vi "MesaurementProcedure.vi"(8 "error in (no error)":errorcluster) -> (0 "error out":errorcluster)   [LabVIEW 2013]
uses:
  Utilities/controls/ctlSeqFNs_PI_SysNr.ctl
  Camera/lib/atmcd32d.llb/Error Code Enum typedef.ctl
  <vilib>/DAQmx/write.llb/DAQmx Write (Analog DBL 1Chan 1Samp).vi
  <vilib>/DAQmx/read.llb/DAQmx Read (Analog DBL 1Chan 1Samp).vi
  Variables/GlobalSetGetPixelOfRoi.vi
  Variables/GlobalSetConfigurationPhysikalInstruments.vi
  Variables/ccdChipPixels.vi
  Variables/GlobalSetGetConfigureCamera.vi
  Variables/SavPath.vi
  Variables/GlobalDevice.vi
  Variables/MesaurementModus.vi
  Variables/ScanrangeY.vi
  Variables/ScanrangeX.vi
  <vilib>/DAQmx/create/channels.llb/DAQmx Create Channel (CO-Pulse Generation-Frequency).vi
  <vilib>/DAQmx/configure/trigger.llb/DAQmx Start Trigger (Digital Edge).vi
  <vilib>/DAQmx/configure/timing.llb/DAQmx Timing (Implicit).vi
  <vilib>/DAQmx/create/channels.llb/DAQmx Create Channel (AI-Voltage-Basic).vi
  <vilib>/DAQmx/create/channels.llb/DAQmx Create Channel (AO-Voltage-Basic).vi
  <vilib>/DAQmx/miscellaneous.llb/DAQmx Fill In Error Info.vi
  Variables/GlobalMesaurementOut.vi
  <resource>/objmgr/daqmx.rc
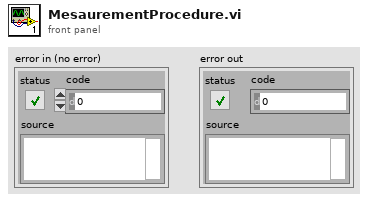
[diagram p1: front panel]
types:
  T1 = typedef "ctlSeqFNs_PI_SysNr.ctl" = enum16{"Zero", "E517", "E710"}
  T2 = typedef "Error Code Enum typedef.ctl" = enum32{"N/A (0)", "DRV_ERROR_CODES", "DRV_SUCCESS", "DRV_VXDNOTINSTALLED", "DRV_ERROR_SCAN", "DRV_ERROR_CHECK_SUM", "DRV_ERROR_FILELOAD", "DRV_UNKNOWN_FUNC", "DRV_ERROR_VXD_INIT", "DRV_ERROR_ADDRESS", "DRV_ERROR_PAGELOCK", "DRV_ERROR_PAGEUNLOCK", "DRV_ERROR_BOARDTEST", "DRV_ERROR_ACK", "DRV_ERROR_UP_FIFO", "DRV_ERROR_PATTERN", "N/A (16)", "DRV_ACQUISITION_ERRORS", "DRV_ACQ_BUFFER", "DRV_ACQ_DOWNFIFO_FULL", "DRV_PROC_UNKONWN_INSTRUCTION", "DRV_ILLEGAL_OP_CODE", "DRV_KINETIC_TIME_NOT_MET", "DRV_ACCUM_TIME_NOT_MET", "DRV_NO_NEW_DATA", "N/A (25)", "DRV_SPOOLERROR", "N/A (27)", "N/A (28)", "N/A (29)", "N/A (30)", "N/A (31)", "N/A (32)", "DRV_TEMPERATURE_CODES", "DRV_TEMPERATURE_OFF", "DRV_TEMPERATURE_NOT_STABILIZED", "DRV_TEMPERATURE_STABILIZED", "DRV_TEMPERATURE_NOT_REACHED", "DRV_TEMPERATURE_OUT_RANGE", "DRV_TEMPERATURE_NOT_SUPPORTED", "DRV_TEMPERATURE_DRIFT", "N/A (41)", "N/A (42)", "N/A (43)", "N/A (44)", "N/A (45)", "N/A (46)", "N/A (47)", "N/A (48)", "DRV_GENERAL_ERRORS", "DRV_INVALID_AUX", "DRV_COF_NOTLOADED", "DRV_FPGAPROG", "DRV_FLEXERROR", "DRV_GPIBERROR", "N/A (55)", "N/A (56)", "N/A (57)", "N/A (58)", "N/A (59)", "N/A (60)", "N/A (61)", "N/A (62)", "N/A (63)", "DRV_DATATYPE", "DRV_DRIVER_ERRORS", "DRV_P1INVALID", "DRV_P2INVALID", "DRV_P3INVALID", "DRV_P4INVALID", "DRV_INIERROR", "DRV_COFERROR", "DRV_ACQUIRING", "DRV_IDLE", "DRV_TEMPCYCLE", "DRV_NOT_INITIALIZED", "DRV_P5INVALID", "DRV_P6INVALID", "DRV_INVALID_MODE", "DRV_INVALID_FILTER", "DRV_I2CERRORS", "DRV_I2CDEVNOTFOUND", "DRV_I2CTIMEOUT", "DRV_P7INVALID", "N/A (84)", "N/A (85)", "N/A (86)", "N/A (87)", "N/A (88)", "N/A (89)", "DRV_IOCERROR", "DRV_VRMVERSIONERROR"}
  T3 = cluster{"Conn. Axes scanner[0]":string, "Conn. Axes scanner[1]":string, "Conn. Axes scanner[2]":string}
  T4 = enum16{"open", "replace", "create", "open or create", "replace or create", "replace or create with confirmation"}
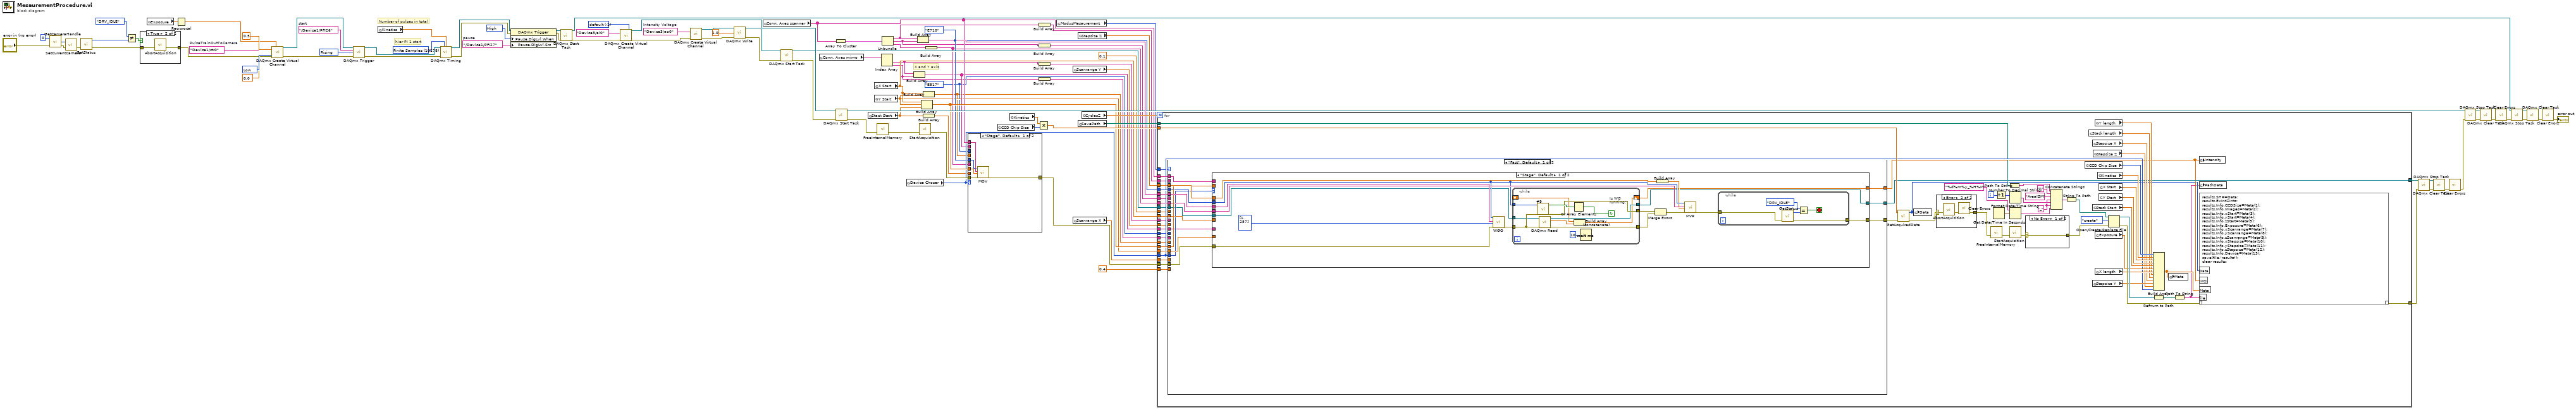
[diagram p0: block diagram]
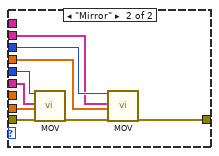
[diagram p2: hidden frame]
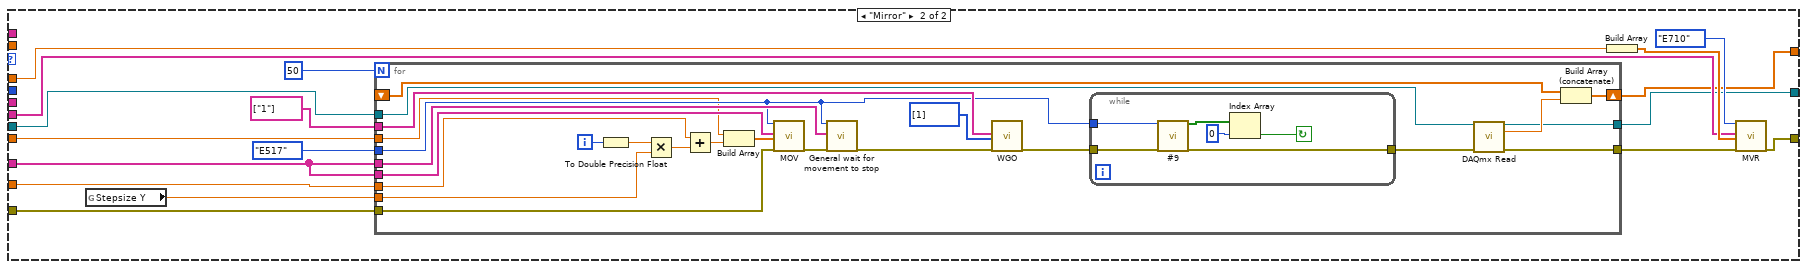
[diagram p3: hidden frame]
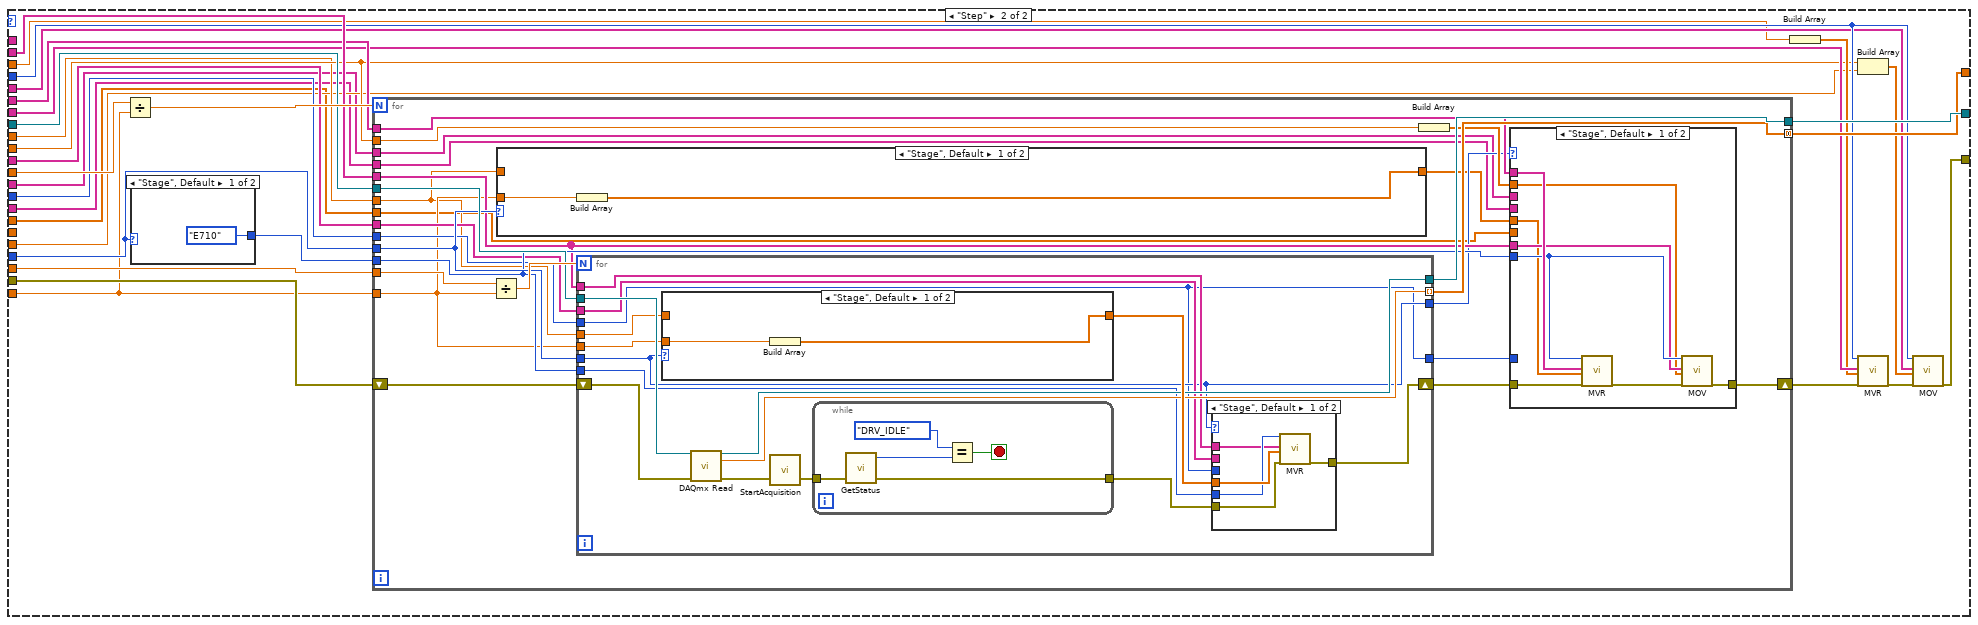
[diagram p4: hidden frame]
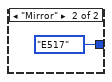
[diagram p5: hidden frame]
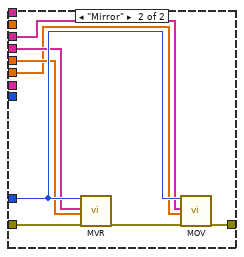
[diagram p6: hidden frame]
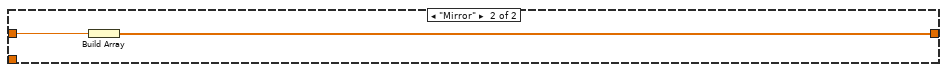
[diagram p7: hidden frame]
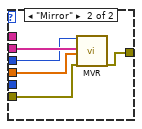
[diagram p8: hidden frame]
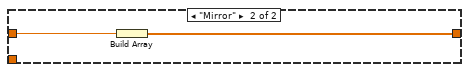
[diagram p9: hidden frame]
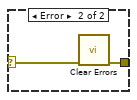
[diagram p11: hidden frame]
diagram:
  w10 = tag "/Device1/PFI26"  # start
  w11 = tag "/Device1/PFI27"  # pause
  w16 = 10192 items=["High"=10192, "Low"=10214] ("Pause.DigLvl.When")
  w21 = 10280 items=["Rising"=10280, "Falling"=10171] ("Trigger Edge")
  w17 = tag "Device1/ctr0"  # PulseTrainOutToCamera
  w27 = 10214 items=["High"=10192, "Low"=10214] ("Idle State")
  w28 = 10178 items=["Finite Samples"=10178, "Continuous Samples"=10123] ("sample mode")
  w36 = ctlSeqFNs_PI_SysNr."E517" ("DeviceNr.")
  w76 = tag "Device3/ao0"  # Intensity Voltage
  w78 = -1 items=["default"=-1, "RSE"=10083, "NRSE"=10078, "Differential"=10106, "Pseudodifferential"=12529] ("input terminal configuration")
  w51 = ctlSeqFNs_PI_SysNr."E710" ("DeviceNr.")
  # "Number of pulses in total"
  # "hier PI 1 start"
  # "X and Y axis"
  n1 = call "GetCameraHandle.vi"("error in (no error)"="error in (no error)", "cameraIndex"=0) -> ("error out"=w86:errorcluster, "cameraHandle"=w85:i32)  [unwired: 1 in, 1 out]
  n2 = call "SetCurrentCamera.vi"("error in (no error)"=w86, "cameraHandle"=w85) -> ("error out"=w87:errorcluster)  [unwired: 1 out]
  n3 = call "GetStatus.vi"("error in (no error)"=w87) -> ("error out"=w92:errorcluster, "status"=w89:T2)  [unwired: 2 in, 1 out]
  n4 = Not Equal?(x=Error_Code_Enum_typedef."DRV_IDLE" ("status"), y=w89) -> (x != y?=w91:bool)
  n5 = case shown="True" w91 {
    tunnel: w92 -> [w99 w101]
    tunnel: [w99 w100] -> w19
    frame False {
    }
    frame True {
      n6 = call "AbortAcquisition.vi"("error in (no error)"=w101) -> ("error out"=w100:errorcluster)  [unwired: 1 in, 1 out]
    }
  }
  n7 = global read "GlobalSetGetConfigureCamera.vi" "Exposure"() -> (w2:sgl)
  n8 = Reciprocal(x=w2) -> (1/x=w3:sgl)
  n9 = call-poly <vilib>:"DAQmx Create Virtual Channel.vi"("frequency"=w3, "duty cycle"=0.5 ("Duty Cycle"), "counter"=w17, "error in"=w19, "idle state"=w27, "initial delay"=0.0) -> ("task out"=w24:refnum<k21>, "error out"=w22:errorcluster)  [unwired: 8 in]
  n10 = call-poly <vilib>:"DAQmx Trigger.vi"("task/channels in"=w24, "source"=w10, "edge"=w21, "error in"=w22) -> ("task out"=w20:refnum<k21>, "error out"=w23:errorcluster)  [unwired: 10 in]
  n11 = global read "GlobalSetGetConfigureCamera.vi" "Kinetics"() -> (w1:sgl)
  n12 = call-poly <vilib>:"DAQmx Timing.vi"("task/channels in"=w20, "sample mode"=w28, "samples per channel"=w1, "error in"=w23) -> ("task out"=w13:refnum<k21>, "error out"=w15:errorcluster)  [unwired: 10 in]
  n13 = property class="DAQmx Trigger"(reference=w13, error in=w15, "Pause.DigLvl.When"=w16, "Pause.DigLvl.Src"=w11) -> (reference out=w12:refnum<k21>, error out=w14:errorcluster)
  n14 = call <vilib>:"DAQmx Start Task.vi"("task/channels in"=w12, "error in"=w14) -> ("task out"=w4:refnum<k21>, "error out"=w18:errorcluster)  [unwired: 12 in]
  n15 = call-poly <vilib>:"DAQmx Create Virtual Channel.vi"("input terminal configuration"=w78, "physical channels"=tag "Device3/ai0", "error in"=w18) -> ("task out"=w67:refnum<k21>, "error out"=w68:errorcluster)  [unwired: 11 in]
  n16 = call-poly <vilib>:"DAQmx Create Virtual Channel.vi"("physical channels"=w76, "error in"=w68) -> ("task out"=w75:refnum<k21>, "error out"=w77:errorcluster)  [unwired: 12 in]
  n17 = call-poly <vilib>:"DAQmx Write.vi"("task/channels in"=w75, "data"=1.0, "error in"=w77) -> ("task out"=w71:refnum<k21>, "error out"=w73:errorcluster)  [unwired: 10 in, 1 out]
  n18 = global read "GlobalSetConfigurationPhysikalInstruments.vi" "Conn. Axes scanner"() -> (w52:string[])
  n19 = call <vilib>:"DAQmx Start Task.vi"("task/channels in"=w67, "error in"=w73) -> ("task out"=w66:refnum<k21>, "error out"=w72:errorcluster)  [unwired: 12 in]
  n20 = global read "GlobalSetConfigurationPhysikalInstruments.vi" "Conn. Axes mirrro"() -> (w50:string[])
  n21 = Array To Cluster(array=w52) -> (cluster=w84:T3)
  n22 = call <vilib>:"DAQmx Start Task.vi"("task/channels in"=w71, "error in"=w72) -> ("task out"=w61:refnum<k21>, "error out"=w70:errorcluster)  [unwired: 12 in]
  n23 = global read "GlobalSetGetPixelOfRoi.vi" "Stack Start"() -> (w44:dbl)
  n24 = global read "GlobalSetGetPixelOfRoi.vi" "X Start"() -> (w40:dbl)
  n25 = global read "GlobalSetGetPixelOfRoi.vi" "Y Start"() -> (w39:dbl)
  n26 = call "FreeInternalMemory.vi"("error in (no error)"=w70) -> ("error out"=w93:errorcluster)  [unwired: 1 in, 1 out]
  n27 = Index Array(array=w50) -> (element #1=w38:string, element #2=w34:string)  [unwired: 2 in]
  n28 = Unbundle(w84) -> ("Conn. Axes scanner[0]"=w49:string, "Conn. Axes scanner[1]"=w47:string, "Conn. Axes scanner[2]"=w83:string)
  n29 = global read "GlobalDevice.vi" "Device Choser"() -> (w45:enum32{"Stage", "Mirror"})
  n30 = Build Array(w38, w34) -> (w41:string[])
  n31 = Build Array(w49, w47) -> (w82:string[])
  n32 = call "StartAcquisition.vi"("error in (no error)"=w93) -> ("error out"=w54:errorcluster)  [unwired: 1 in, 1 out]
  n33 = Build Array(w40, w39, w44) -> (w53:dbl[])
  n34 = Build Array(w40, w39) -> (w32:dbl[])
  n35 = Build Array(w44) -> (w43:dbl[])
  n36 = Build Array(w83) -> (w42:string[])
  n37 = case shown="\"Stage\", Default" w45 {
    tunnel: [w106 w115] -> w55
    tunnel: w54 -> [w105 w113]
    tunnel: w53 -> [w104 _]
    tunnel: w52 -> [w103 _]
    tunnel: w51 -> [w102 w110]
    tunnel: w43 -> [_ w112]
    tunnel: w42 -> [_ w111]
    tunnel: w36 -> [_ w109]
    tunnel: w41 -> [_ w108]
    tunnel: w32 -> [_ w107]
    frame "Stage", Default {
      n38 = call "MOV.vi"("System no."=w102, "Axes to move"=w103, "Position values"=w104, "error in"=w105) -> ("error out"=w106:errorcluster)  [unwired: 1 in, 14 out]
    }
    frame "Mirror" {
      n39 = call "MOV.vi"("System no."=w110, "Axes to move"=w111, "Position values"=w112, "error in"=w113) -> ("error out"=w114:errorcluster)  [unwired: 1 in, 14 out]
      n40 = call "MOV.vi"("System no."=w109, "Axes to move"=w108, "Position values"=w107, "error in"=w114) -> ("error out"=w115:errorcluster)  [unwired: 1 in, 14 out]
    }
  }
  n41 = global read "ccdChipPixels.vi" "CCD Chip Size"() -> (w96:i32)
  n42 = global read "GlobalSetGetConfigureCamera.vi" "Kinetics"() -> (w97:sgl)
  n43 = Multiply(x=w97, y=w96) -> (x*y=w94:sgl)
  n44 = Build Array(w49) -> (w48:string[])
  n45 = Build Array(w47) -> (w46:string[])
  n46 = Build Array(w38) -> (w37:string[])
  n47 = Build Array(w34) -> (w33:string[])
  n48 = global read "MesaurementModus.vi" "ModusMesaurement"() -> (w30:enum32{"Fast", "Step"})
  n49 = global read "ScanrangeY.vi" "Scanrange Y"() -> (w56:dbl)
  n50 = global read "ScanrangeX.vi" "Scanrange X"() -> (w57:dbl)
  n51 = global read "GlobalSetGetPixelOfRoi.vi" "Stepsize Z"() -> (w31:dbl)
  n52 = global read "SavPath.vi" "SavePath"() -> (w95:path)
  n53 = global read "GlobalSetGetPixelOfRoi.vi" "CyclesZ"() -> (w98:dbl)
  n54 = for {
    N: w98 -> [_]
    tunnel: w52 -> [w180]
    tunnel: w31 -> [w179]
    tunnel: w82 -> [w178]
    tunnel: w53 -> [w177]
    tunnel: w42 -> [w176]
    tunnel: w51 -> [w175]
    tunnel: w94 -> [w174]
    tunnel: w95 -> [w120]
    tunnel: [w173] -> w63
    tunnel: w55 -> [w172]
    tunnel: w39 -> [w139]
    tunnel: w40 -> [w138]
    tunnel: w45 -> [w136]
    tunnel: w66 -> [w134]
    tunnel: [w133] -> w65
    tunnel: w30 -> [w132]
    tunnel: w57 -> [w130]
    tunnel: w56 -> [w131]
    tunnel: w41 -> [w129]
    tunnel: w48 -> [w128]
    tunnel: w46 -> [w127]
    tunnel: w37 -> [w126]
    tunnel: w36 -> [w125]
    tunnel: 0.1 -> [w124]
    tunnel: 0.4 -> [w123]
    tunnel: w33 -> [w122]
    tunnel: w32 -> [w121]
    i -> [w137]
    w155 = "_" ("string")
    n55 = case shown="\"Fast\", Default" w132 {
      tunnel: w180 -> [w195 _]
      tunnel: w179 -> [w194 w276]
      tunnel: w178 -> [w193 w287]
      tunnel: w177 -> [w192 _]
      tunnel: w176 -> [w191 w292]
      tunnel: w175 -> [w190 w288]
      tunnel: w172 -> [w189 w301]
      tunnel: [w188 w289] -> w171
      tunnel: w139 -> [w187 w280]
      tunnel: w138 -> [w186 w285]
      tunnel: w136 -> [w185 w295]
      tunnel: w134 -> [w184 w299]
      tunnel: [w183 w298] -> w133
      tunnel: [w182 w297] -> w119
      tunnel: w131 -> [_ w300]
      tunnel: w130 -> [_ w303]
      tunnel: w129 -> [w181 w278]
      tunnel: w128 -> [_ w294]
      tunnel: w127 -> [_ w293]
      tunnel: w126 -> [_ w284]
      tunnel: w125 -> [_ w283]
      tunnel: w124 -> [_ w282]
      tunnel: w123 -> [_ w281]
      tunnel: w122 -> [_ w279]
      tunnel: w121 -> [_ w277]
      frame "Fast", Default {
        n56 = case shown="\"Stage\", Default" w185 {
          tunnel: w195 -> [_ _]
          tunnel: w194 -> [w211 w236]
          tunnel: w193 -> [w210 _]
          tunnel: w192 -> [_ _]
          tunnel: w191 -> [w209 w234]
          tunnel: w190 -> [w208 _]
          tunnel: w189 -> [w196 w239]
          tunnel: [w203 w238] -> w188
          tunnel: w187 -> [_ w241]
          tunnel: w186 -> [_ w240]
          tunnel: [w199 w232] -> w182
          tunnel: w184 -> [w198 w231]
          tunnel: [w197 w230] -> w183
          tunnel: w181 -> [_ w229]
          frame "Stage", Default {
            n57 = call "WGO.vi"("System no."=w208, "Affected axes"=w210, "WGO Parameter"=i32[] [1, 257], "error in"=w196) -> ("error out"=w206:errorcluster)  [unwired: 15 out]
            n58 = while {
              tunnel: w208 -> [w224]
              tunnel: [w225] -> w201
              tunnel: w206 -> [w223]
              tunnel: [w222] -> w202
              tunnel: w198 -> [w221]
              tunnel: [w220] -> w197
              shift-right: [w217] -> w199
              shift-left: _ -> [w219]
              stop <- w227 continue-if-true
              # "Is WG\nrunning?"
              n59 = call "#9.vi"("System no."=w224, "error in"=w223) -> ("WG running?"=w228:bool[], "error out"=w225:errorcluster)  [unwired: 16 out]
              n60 = call-poly <vilib>:"DAQmx Read.vi"("task/channels in"=w221, "error in"=w223) -> ("task out"=w220:refnum<k21>, "data"=w218:dbl, "error out"=w222:errorcluster)  [unwired: 11 in]
              n61 = Or Array Elements(Boolean array=w228) -> (logical OR=w227:bool)
              n62 = Build Array (concatenate)(w219, w218) -> (w217:dbl[])
              n63 = Wait (ms)(milliseconds to wait=u32 10) -> ()  [unwired: 1 out]
            }
            n64 = Merge Errors(w201, w202) -> (w200:errorcluster)
            n65 = Build Array(w211) -> (w205:dbl[])
            n66 = call "MVR.vi"("System no."=w208, "Axes to move"=w209, "Position values"=w205, "error in"=w200) -> ("error out"=w204:errorcluster)  [unwired: 1 in, 14 out]
            n67 = while {
              tunnel: w204 -> [w212]
              tunnel: [w214] -> w203
              stop <- w213 stop-if-true
              n68 = call "GetStatus.vi"("error in (no error)"=w212) -> ("error out"=w214:errorcluster, "status"=w215:T2)  [unwired: 2 in, 1 out]
              n69 = Equal?(x=Error_Code_Enum_typedef."DRV_IDLE" ("status"), y=w215) -> (x = y?=w213:bool)
            }
          }
          frame "Mirror" {
            n70 = global read "GlobalSetGetPixelOfRoi.vi" "Stepsize Y"() -> (w244:dbl)
            n71 = for {
              N: 50 -> [_]
              tunnel: w239 -> [w262]
              tunnel: w229 -> [w261]
              tunnel: w229 -> [w260]
              tunnel: string[] ["1"] ("Affected axes") -> [w257]
              tunnel: ctlSeqFNs_PI_SysNr."E517" ("DeviceNr.") -> [w256]
              tunnel: w244 -> [w255]
              tunnel: w241 -> [w254]
              tunnel: w240 -> [w253]
              tunnel: [w251] -> w233
              shift-right: [w248] -> w232
              shift-left: _ -> [w250]
              tunnel: w231 -> [w247]
              tunnel: [w246] -> w230
              i -> [w266]
              n72 = To Double Precision Float(number=w266) -> (double precision float=w267:dbl)
              n73 = Multiply(x=w267, y=w255) -> (x*y=w258:dbl)
              n74 = Add(x=w254, y=w258) -> (x+y=w265:dbl)
              n75 = Build Array(w253, w265) -> (w264:dbl[])
              n76 = call "MOV.vi"("System no."=w256, "Axes to move"=w261, "Position values"=w264, "error in"=w262) -> ("error out"=w263:errorcluster)  [unwired: 1 in, 14 out]
              n77 = call "General wait for movement to stop.vi"("System no."=w256, "Axes to wait for"=w260, "error in"=w263) -> ("error out"=w259:errorcluster)  [unwired: 5 in, 11 out]
              n78 = call "WGO.vi"("Affected axes"=w257, "WGO Parameter"=i32[] [1] ("Generator ID"), "error in"=w259) -> ("error out"=w268:errorcluster)  [unwired: 1 in, 15 out]
              n79 = while {
                tunnel: w268 -> [w270]
                tunnel: [w275] -> w252
                tunnel: w256 -> [w271]
                stop <- w272 continue-if-true
                n80 = call "#9.vi"("System no."=w271, "error in"=w270) -> ("WG running?"=w274:bool[], "error out"=w275:errorcluster)  [unwired: 16 out]
                n81 = Index Array(array=w274, index=0) -> (element=w272:bool)
              }
              n82 = call-poly <vilib>:"DAQmx Read.vi"("task/channels in"=w247, "error in"=w252) -> ("task out"=w246:refnum<k21>, "data"=w249:dbl, "error out"=w251:errorcluster)  [unwired: 11 in]
              n83 = Build Array (concatenate)(w250, w249) -> (w248:dbl[])
            }
            n84 = Build Array(w236) -> (w235:dbl[])
            n85 = call "MVR.vi"("System no."=ctlSeqFNs_PI_SysNr."E710" ("DeviceNr."), "Axes to move"=w234, "Position values"=w235, "error in"=w233) -> ("error out"=w238:errorcluster)  [unwired: 1 in, 14 out]
          }
        }
      }
      frame "Step" {
        n86 = Divide(x=w300, y=w281) -> (x/y=w304:dbl)
        n87 = case shown="\"Stage\", Default" w295 {
          tunnel: [ctlSeqFNs_PI_SysNr."E710" ("DeviceNr.") ctlSeqFNs_PI_SysNr."E517" ("DeviceNr.")] -> w296
          frame "Stage", Default {
          }
          frame "Mirror" {
          }
        }
        n88 = for {
          N: w304 -> [_]
          tunnel: w303 -> [w329]
          tunnel: w281 -> [w314]
          shift-right: [w321] -> w302
          shift-left: w301 -> [w328]
          tunnel: w299 -> [w326]
          tunnel: [w325] -> w298
          tunnel: [w324] -> w297 mode=concatenating
          tunnel: w296 -> [w320]
          tunnel: w295 -> [w323]
          tunnel: w294 -> [w319]
          tunnel: w293 -> [w322]
          tunnel: w285 -> [w318]
          tunnel: w284 -> [w316]
          tunnel: w283 -> [w315]
          tunnel: w282 -> [w313]
          tunnel: w279 -> [w309]
          tunnel: w278 -> [w308]
          tunnel: w277 -> [w307]
          n89 = Divide(x=w329, y=w314) -> (x/y=w330:dbl)
          n90 = case shown="\"Stage\", Default" w323 {
            tunnel: w314 -> [w348 _]
            tunnel: w313 -> [_ w350]
            tunnel: [w347 w349] -> w310
            frame "Stage", Default {
              n91 = Build Array(w348) -> (w347:dbl[])
            }
            frame "Mirror" {
              n92 = Build Array(w350) -> (w349:dbl[])
            }
          }
          n93 = for {
            N: w330 -> [_]
            shift-right: [w366] -> w327
            shift-left: w328 -> [w363]
            tunnel: w326 -> [w364]
            tunnel: [w359] -> w325
            tunnel: [w358] -> w324 mode=indexing
            tunnel: w320 -> [w357]
            tunnel: w323 -> [w352]
            tunnel: w319 -> [w356]
            tunnel: w316 -> [w355]
            tunnel: w315 -> [w351]
            tunnel: w314 -> [w354]
            tunnel: w313 -> [w353]
            tunnel: [w352] -> w312
            tunnel: [w351] -> w311
            n94 = case shown="\"Stage\", Default" w352 {
              tunnel: [w378 w380] -> w365
              tunnel: w354 -> [w377 _]
              tunnel: w353 -> [_ w379]
              frame "Stage", Default {
                n95 = Build Array(w377) -> (w378:dbl[])
              }
              frame "Mirror" {
                n96 = Build Array(w379) -> (w380:dbl[])
              }
            }
            n97 = call-poly <vilib>:"DAQmx Read.vi"("task/channels in"=w364, "error in"=w363) -> ("task out"=w359:refnum<k21>, "data"=w358:dbl, "error out"=w362:errorcluster)  [unwired: 11 in]
            n98 = call "StartAcquisition.vi"("error in (no error)"=w362) -> ("error out"=w361:errorcluster)  [unwired: 1 in, 1 out]
            n99 = while {
              tunnel: w361 -> [w381]
              tunnel: [w383] -> w360
              stop <- w382 stop-if-true
              n100 = call "GetStatus.vi"("error in (no error)"=w381) -> ("error out"=w383:errorcluster, "status"=w384:T2)  [unwired: 2 in, 1 out]
              n101 = Equal?(x=Error_Code_Enum_typedef."DRV_IDLE" ("status"), y=w384) -> (x = y?=w382:bool)
            }
            n102 = case shown="\"Stage\", Default" w352 {
              tunnel: [w371 w372] -> w366
              tunnel: w365 -> [w370 w373]
              tunnel: w360 -> [w369 w376]
              tunnel: w357 -> [w368 _]
              tunnel: w356 -> [w367 _]
              tunnel: w355 -> [_ w375]
              tunnel: w351 -> [_ w374]
              frame "Stage", Default {
                n103 = call "MVR.vi"("System no."=w368, "Axes to move"=w367, "Position values"=w370, "error in"=w369) -> ("error out"=w371:errorcluster)  [unwired: 1 in, 14 out]
              }
              frame "Mirror" {
                n104 = call "MVR.vi"("System no."=w374, "Axes to move"=w375, "Position values"=w373, "error in"=w376) -> ("error out"=w372:errorcluster)  [unwired: 1 in, 14 out]
              }
            }
          }
          n105 = Build Array(w318) -> (w317:dbl[])
          n106 = case shown="\"Stage\", Default" w312 {
            tunnel: w327 -> [w338 w344]
            tunnel: w322 -> [w337 _]
            tunnel: [w335 w345] -> w321
            tunnel: w320 -> [w334 _]
            tunnel: w319 -> [w333 _]
            tunnel: w317 -> [w332 _]
            tunnel: w311 -> [_ w343]
            tunnel: w310 -> [w331 w342]
            tunnel: w309 -> [_ w341]
            tunnel: w308 -> [_ w340]
            tunnel: w307 -> [_ w339]
            frame "Stage", Default {
              n107 = call "MVR.vi"("System no."=w334, "Axes to move"=w337, "Position values"=w331, "error in"=w338) -> ("error out"=w336:errorcluster)  [unwired: 1 in, 14 out]
              n108 = call "MOV.vi"("System no."=w334, "Axes to move"=w333, "Position values"=w332, "error in"=w336) -> ("error out"=w335:errorcluster)  [unwired: 1 in, 14 out]
            }
            frame "Mirror" {
              n109 = call "MVR.vi"("System no."=w343, "Axes to move"=w341, "Position values"=w342, "error in"=w344) -> ("error out"=w346:errorcluster)  [unwired: 1 in, 14 out]
              n110 = call "MOV.vi"("System no."=w343, "Axes to move"=w340, "Position values"=w339, "error in"=w346) -> ("error out"=w345:errorcluster)  [unwired: 1 in, 14 out]
            }
          }
        }
        n111 = Build Array(w276) -> (w291:dbl[])
        n112 = Build Array(w285, w280) -> (w286:dbl[])
        n113 = call "MVR.vi"("System no."=w288, "Axes to move"=w292, "Position values"=w291, "error in"=w302) -> ("error out"=w290:errorcluster)  [unwired: 1 in, 14 out]
        n114 = call "MOV.vi"("System no."=w288, "Axes to move"=w287, "Position values"=w286, "error in"=w290) -> ("error out"=w289:errorcluster)  [unwired: 1 in, 14 out]
      }
    }
    n115 = call "GetAcquiredData.vi"("error in (no error)"=w171, "size"=w174) -> ("error out"=w135:errorcluster, "array"=w117:i32[])  [unwired: 1 in, 1 out]
    n116 = global write "GlobalMesaurementOut.vi" "Data"(w117) -> ()
    n117 = case shown="Error" w135 {
      selector: w135 -> [w386 w387]
      tunnel: [w386 w389] -> w169
      frame No Error {
      }
      frame Error {
        n118 = call "AbortAcquisition.vi"("error in (no error)"=w387) -> ("error out"=w388:errorcluster)  [unwired: 1 in, 1 out]
        n119 = call <vilib>:"Clear Errors.vi"("error in (no error)"=w388) -> ("error out"=w389:errorcluster)  [unwired: 6 in]
      }
    }
    n120 = call "FreeInternalMemory.vi"("error in (no error)"=w169) -> ("error out"=w170:errorcluster)  [unwired: 1 in, 1 out]
    n121 = Get Date/Time In Seconds() -> (seconds since 1Jan1904=w158:timestamp)
    n122 = Increment(x=w137) -> (x+1=w167:i32)
    n123 = Path To String(path=w120) -> (string=w162:string)
    n124 = Number To Decimal String(number=w167) -> (decimal integer string=w159:string)  [unwired: 1 in]
    n125 = Format Date/Time String(time format string (%c)="%d%m%y_%H%M", seconds (now)=w158) -> (date/time string=w156:string)  [unwired: 1 in]
    n126 = call "StartAcquisition.vi"("error in (no error)"=w170) -> ("error out"=w168:errorcluster)  [unwired: 1 in, 1 out]
    n127 = case shown="No Error" w168 {
      selector: w168 -> [w390 w392]
      tunnel: [w390 w391] -> w153
      frame No Error {
      }
      frame Error {
        n128 = call <vilib>:"Clear Errors.vi"("error in (no error)"=w392) -> ("error out"=w391:errorcluster)  [unwired: 6 in]
      }
    }
    n129 = Concatenate Strings(w162, "\\" ("string"), "AreaISM" ("string"), w155, w159, w155, w156) -> (w163:string)
    n130 = String To Path(string=w163) -> (path=w164:path)
    n131 = global read "ccdChipPixels.vi" "CCD Chip Size"() -> (w151:i32)
    n132 = global read "GlobalSetGetPixelOfRoi.vi" "Stack length"() -> (w143:dbl)
    n133 = global read "GlobalSetGetPixelOfRoi.vi" "Stepsize X"() -> (w142:dbl)
    n134 = global read "GlobalSetGetPixelOfRoi.vi" "Stack Start"() -> (w147:dbl)
    n135 = global read "GlobalSetGetPixelOfRoi.vi" "Stepsize Y"() -> (w141:dbl)
    n136 = global read "GlobalSetGetPixelOfRoi.vi" "Stepsize Z"() -> (w140:dbl)
    n137 = global read "GlobalSetGetPixelOfRoi.vi" "Y length"() -> (w144:dbl)
    n138 = global read "GlobalSetGetConfigureCamera.vi" "Exposure"() -> (w146:sgl)
    n139 = global read "GlobalSetGetPixelOfRoi.vi" "X length"() -> (w145:dbl)
    n140 = global read "GlobalSetGetConfigureCamera.vi" "Kinetics"() -> (w150:sgl)
    n141 = global read "GlobalSetGetPixelOfRoi.vi" "X Start"() -> (w149:dbl)
    n142 = global read "GlobalSetGetPixelOfRoi.vi" "Y Start"() -> (w148:dbl)
    n143 = Open/Create/Replace File(file path (use dialog)=w164, error in=w153, operation (0:open)=T4."create") -> (refnum out=w165:refnum<file>, error out=w152:errorcluster)  [unwired: 4 out]
    n144 = Build Array(w151, w150, w149, w148, w147, w146, w145, w144, w143, w142, w141, w140, w136) -> (w118:dbl[])
    n145 = Refnum to Path(1:w165) -> (0:w154:path)
    n146 = global write "GlobalMesaurementOut.vi" "Meta"(w118) -> ()
    n147 = Path To String(path=w154) -> (string=w116:string)
    n148 = global write "GlobalMesaurementOut.vi" "Intensity"(w119) -> ()
    n149 = global write "GlobalMesaurementOut.vi" "PathData"(w116) -> ()
    n150 = script code="results.SHR=Data;\nresults.ExInt=Ints;\nresults.Info.CCDSize=Meta(1);\nresults.Info.Images=Meta(2);\nresults.Info.xStart=Meta(3);\nresults.Info.yStart=Meta(4);\nresults.Info.zStart=Meta(5);\nresults.Info.Exposure=Meta(6);\nresults.Info.xScanrange=Meta(7);\nresults.Info.yScanrange=Meta(8);\nresults.Info.zScanrange=Meta(9);\nresults.Info.xStepsize=Meta(10);\nresults.Info.yStepsize=Meta(11);\nresults.Info.zStepsize=Meta(12);\nresults.Info.Device=Meta(13);\nsave(file,'results');\nclear results;"("??"=w152, "Data"=w117, "Ints"=w119, "Meta"=w118, "file"=w116) -> ("??"=w173:errorcluster)
  }
  n151 = call <vilib>:"DAQmx Stop Task.vi"("task/channels in"=w65, "error in"=w63) -> ("task out"=w64:refnum<k21>, "error out"=w62:errorcluster)  [unwired: 12 in]
  n152 = call <vilib>:"DAQmx Clear Task.vi"("task in"=w64, "error in"=w62) -> ("error out"=w80:errorcluster)  [unwired: 13 in]
  n153 = call <vilib>:"Clear Errors.vi"("error in (no error)"=w80) -> ("error out"=w59:errorcluster)  [unwired: 6 in]
  n154 = call <vilib>:"DAQmx Stop Task.vi"("task/channels in"=w61, "error in"=w59) -> ("task out"=w60:refnum<k21>, "error out"=w58:errorcluster)  [unwired: 12 in]
  n155 = call <vilib>:"DAQmx Clear Task.vi"("task in"=w60, "error in"=w58) -> ("error out"=w69:errorcluster)  [unwired: 13 in]
  n156 = call <vilib>:"Clear Errors.vi"("error in (no error)"=w69) -> ("error out"=w7:errorcluster)  [unwired: 6 in]
  n157 = call <vilib>:"DAQmx Stop Task.vi"("task/channels in"=w4, "error in"=w7) -> ("task out"=w5:refnum<k21>, "error out"=w8:errorcluster)  [unwired: 12 in]
  n158 = call <vilib>:"DAQmx Clear Task.vi"("task in"=w5, "error in"=w8) -> ("error out"=w9:errorcluster)  [unwired: 13 in]
  n159 = call <vilib>:"Clear Errors.vi"("error in (no error)"=w9) -> ("error out"=→"error out":errorcluster)  [unwired: 6 in]
